vi "PRO_Detect Switch Point.vi"(6 "error in (no error)":errorcluster, 7 "Enable":bool, 8 "Drain!Fill":bool, 9 "Fitler TC":dbl=0.9, 10 "Measure N-1":T2={"Ch A   Ohms"=100.0, " Ch B  Ohms"=100.0, "Level OUt"=3.672222222222213}, 11 "Measure N":T2={"Ch A   Ohms"=100.0, " Ch B  Ohms"=200.0, "Level OUt"=3.699999999999991}) -> (0 "ChB Switch":bool=TRUE, 1 "ChA Switch":bool, 2 "XResult":T1=[{"Switched"=FALSE, "In Range"=TRUE, "Index"=1, "Level OUt"=3.699999999999991, " Ch n Ohms"=100.0, "Drain!Fill"=FALSE}, {"Switched"=TRUE, "In Range"=TRUE, "Index"=2, "Level OUt"=3.699999999999991, " Ch n Ohms"=100.0, "Drain!Fill"=FALSE}], 3 "Measure N out":T2={"Ch A   Ohms"=100.0, " Ch B  Ohms"=200.0, "Level OUt"=3.697222222222213}, 4 "error out":errorcluster)   [LabVIEW 2024]
uses:
  Control Definitions/Def Xresult.ctl
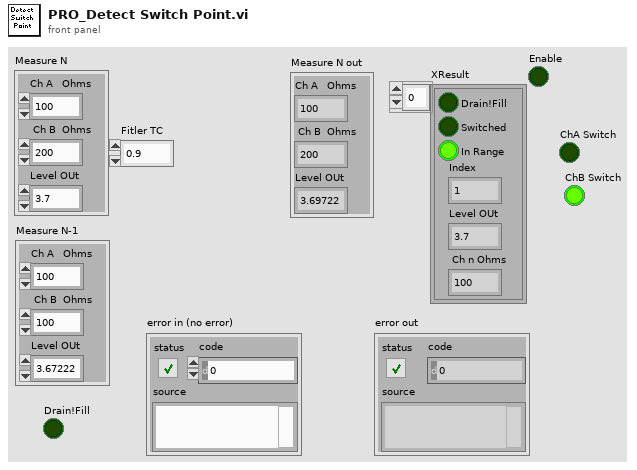
[diagram p1: front panel]
types:
  T1 = typedef "Def Xresult.ctl" = cluster{"Switched":bool, "In Range":bool, "Index":i16, "Level OUt":dbl, " Ch n Ohms":dbl, "Drain!Fill":bool}[]
  T2 = cluster{"Ch A   Ohms":dbl, " Ch B  Ohms":dbl, "Level OUt":dbl}
  T3 = cluster{"XSwitch":bool, "In Range?":bool, "Rindex":i16, "Level OUt":dbl, "Ch A   Ohms":dbl, "Drain!Fill":bool}
  T4 = cluster{"XSwitch":bool, "In Range?":bool, "Rindex":i16, "Level OUt":dbl, " Ch B  Ohms":dbl, "Drain!Fill":bool}
  T5 = cluster{"XSwitch":bool, "In Range?":bool, "Rindex":i16, "Level OUt":dbl, " Ch B  Ohms":dbl, "Drain!Fill":bool}[]
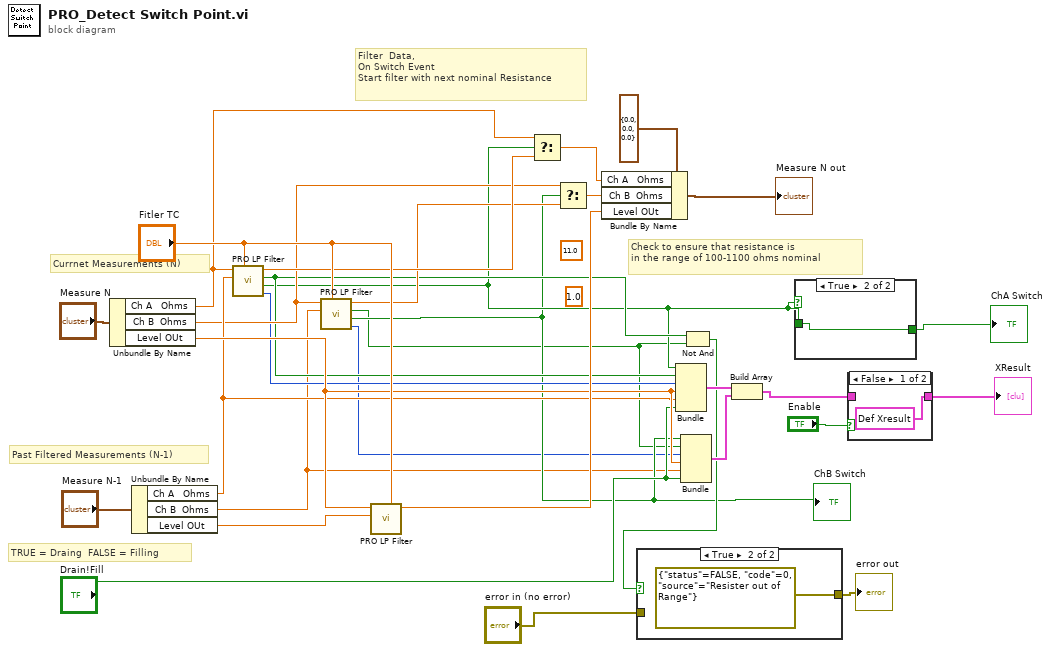
[diagram p0: block diagram]
diagram:
  (unwired) 1.0 ("lower limit")
  (unwired) 11.0 ("upper limit")
  # "TRUE = Draing  FALSE = Filling"
  # "Past Filtered Measurements (N-1)"
  # "Currnet Measurements (N)"
  # "Check to ensure that resistance is \nin the range of 100-1100 ohms nominal"
  # "Filter  Data, \nOn Switch Event\nStart filter with next nominal Resistance"
  n1 = Unbundle By Name("Measure N") -> ("Ch A   Ohms"=w13:dbl, "Ch B  Ohms"=w12:dbl, "Level OUt"=w16:dbl)
  n2 = Unbundle By Name("Measure N-1") -> ("Ch A   Ohms"=w15:dbl, "Ch B  Ohms"=w5:dbl, "Level OUt"=w25:dbl)
  n3 = call "PRO LP Filter.vi"("Fitler TC"="Fitler TC", "In N -1"=w15, "In N"=w13) -> ("Rindex"=w10:i16, "XSwitch"=w9:bool, "In Range?"=w11:bool, "Filtered Out"=w22:dbl)  [unwired: 5 in]
  n4 = call "PRO LP Filter.vi"("Fitler TC"="Fitler TC", "In N -1"=w5, "In N"=w12) -> ("Rindex"=w7:i16, "XSwitch"=w8:bool, "In Range?"=w6:bool, "Filtered Out"=w20:dbl)  [unwired: 5 in]
  "ChB Switch" <- w8
  n5 = call "PRO LP Filter.vi"("Fitler TC"="Fitler TC", "In N -1"=w25, "In N"=w16) -> ("Filtered Out"=w18:dbl)  [unwired: 5 in, 3 out]
  n6 = Select(t=w13, s=w9, f=w22) -> (s? t:f=w21:dbl)
  n7 = Select(t=w12, s=w8, f=w20) -> (s? t:f=w19:dbl)
  n8 = Bundle By Name(cluster=T2 {"Ch A   Ohms"=0.0, " Ch B  Ohms"=0.0, "Level OUt"=0.0} ("Cluster N"), "Ch A   Ohms"=w21, "Ch B  Ohms"=w19, "Level OUt"=w18) -> (→"Measure N out":T2)
  n9 = Bundle("XSwitch"=w9, "In Range?"=w11, "Rindex"=w10, "Level OUt"=w16, "Ch A   Ohms"=w15, "Drain!Fill"="Drain!Fill") -> (w31:T3)  [unwired: 1 in]
  n10 = Bundle("XSwitch"=w8, "In Range?"=w6, "Rindex"=w7, "Level OUt"=w16, "Ch B  Ohms"=w5, "Drain!Fill"="Drain!Fill") -> (w30:T4)  [unwired: 1 in]
  n11 = Not And(1:w6, 2:w11) -> (0:w27:bool)
  n12 = case shown="True" w27 {
    tunnel: "error in (no error)" -> [w33 _]
    tunnel: [w33 errorcluster {"status"=FALSE, "code"=0, "source"="Resister out of Range"} ("error out")] -> w28
    frame False {
    }
    frame True {
    }
  }
  "error out" <- w28
  n13 = Build Array(w31, w30) -> (w2:T5)
  n14 = case shown="True" w9 {
    selector: w9 -> [w35 _]
    tunnel: w9 -> [_ w36]
    tunnel: [w35 w36] -> w4
    frame False {
    }
    frame True {
    }
  }
  "ChA Switch" <- w4
  n15 = case shown="False" "Enable" {
    tunnel: [T1 [{"Switched"=FALSE, "In Range"=TRUE, "Index"=1, "Level OUt"=3.699999999999991, " Ch n Ohms"=100.0, "Drain!Fill"=FALSE}, {"Switched"=TRUE, "In Range"=TRUE, "Index"=2, "Level OUt"=3.699999999999991, " Ch n Ohms"=100.0, "Drain!Fill"=FALSE}] ("XResult") w38] -> w3
    tunnel: w2 -> [_ w38]
    frame False {
    }
    frame True {
    }
  }
  "XResult" <- w3
